vi "writeToXML.vi"(8 "error in (no error)":errorcluster, 10 "ClassLabel":string, 11 "PointNew in":refnum<class "PointNew.lvclass">) -> (0 "error out":errorcluster, 2 "XML out":string, 3 "PointNew out":refnum<class "PointNew.lvclass">)   [LabVIEW 2022 SP3, in "TCSDataDefinitions.lvlib" / "TCSCommand.lvlib" / "PointingFileCommands.lvlib" / "PointNew.lvclass"]
uses:
  PointNew.lvclass
  PointingFileCommands/PointingFileCommands.lvclass
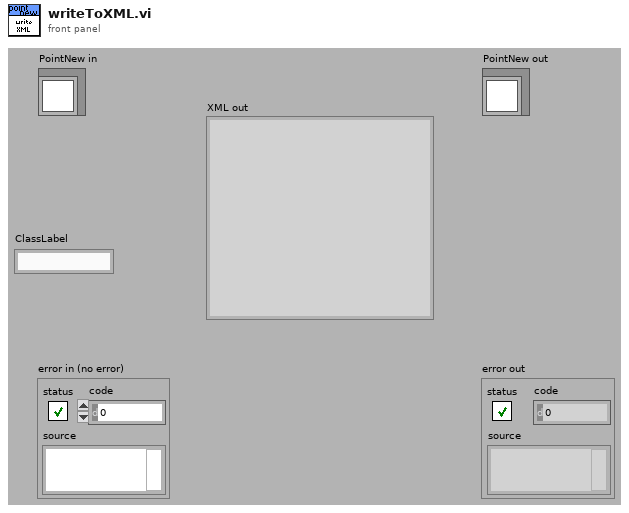
[diagram p1: front panel]
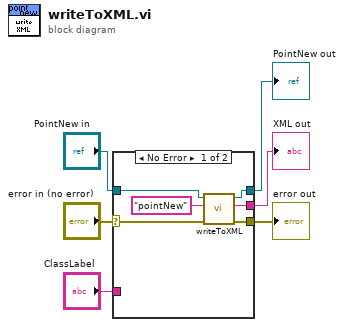
[diagram p0: block diagram]
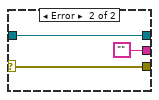
[diagram p2: hidden frame]
diagram:
  n1 = case shown="No Error" "error in (no error)" {
    selector: "error in (no error)" -> [w11 w15]
    tunnel: [w10 w15] -> w5
    tunnel: [w8 w14] -> w3
    tunnel: "PointNew in" -> [w9 w14]
    tunnel: "ClassLabel" -> [_ _]
    tunnel: [w7 ""] -> w1
    frame No Error {
      n2 = call-parent "writeToXML.vi"("error in (no error)"=w11, "ClassLabel"="pointNew", "PointingFileCommands in"=w9) -> ("error out"=w10:errorcluster, "XML out"=w7:string, "PointingFileCommands out"=w8:refnum<class "PointNew.lvclass">)  [unwired: 6 in]
    }
    frame Error {
    }
  }
  "error out" <- w5
  "PointNew out" <- w3
  "XML out" <- w1
